vi "test Initial States Are Activated.vi"(8 "error in (no error)":errorcluster, 11 "TestCase in":refnum<class "Routing and Faulting System Tests.lvclass">) -> (0 "error out":errorcluster, 3 "TestCase out":refnum<class "Routing and Faulting System Tests.lvclass">)   [LabVIEW 2017, in "Routing and Faulting System Tests.lvclass"]
uses:
  Routing and Faulting System Tests.lvclass
  C:/Dev/GitHub/niveristand-custom-device-testing-tools/VeriStandTestCase/VeriStandTestCase.lvclass
  SLSC Switch States.ctl
  Routing and Faulting System Tests.lvclass/Routing and Faulting System Tests.ctl
  <vilib>/NI Veristand/Execution/Workspace/NI VeriStand - Get Single Channel Value.vi
  <vilib>/NI VeriStand/Execution/Workspace/NI_VS Workspace ExecutionAPI.lvlib
  <vilib>/addons/_JKI Toolkits/VI Tester/TestCase.llb/TestCase.lvclass
  C:/Program Files (x86)/National Instruments/LabVIEW 2017/vi.lib/addons/_JKI Toolkits/VI Tester/TestCase.llb/TestCase.lvclass
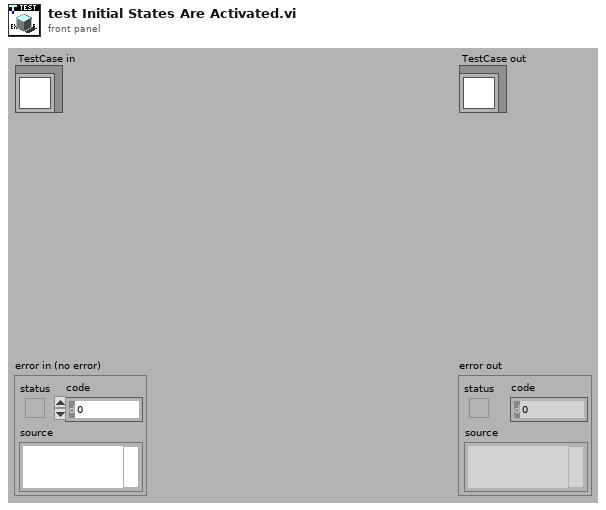
[diagram p1: front panel]
types:
  T1 = typedef "Routing and Faulting System Tests.lvclass/SLSC Switch States.ctl" = cluster{"Channel Load States":cluster{"name":string, "value":i32}[], "Channel Bus States":cluster{"name":string, "value":i32}[], "Channel Pair States":cluster{"name":string, "value":i32}[]}
  T2 = typedef "NI_VS Workspace ExecutionAPI.lvlib/WorkspaceAPI.ctl" = refnum<k24>
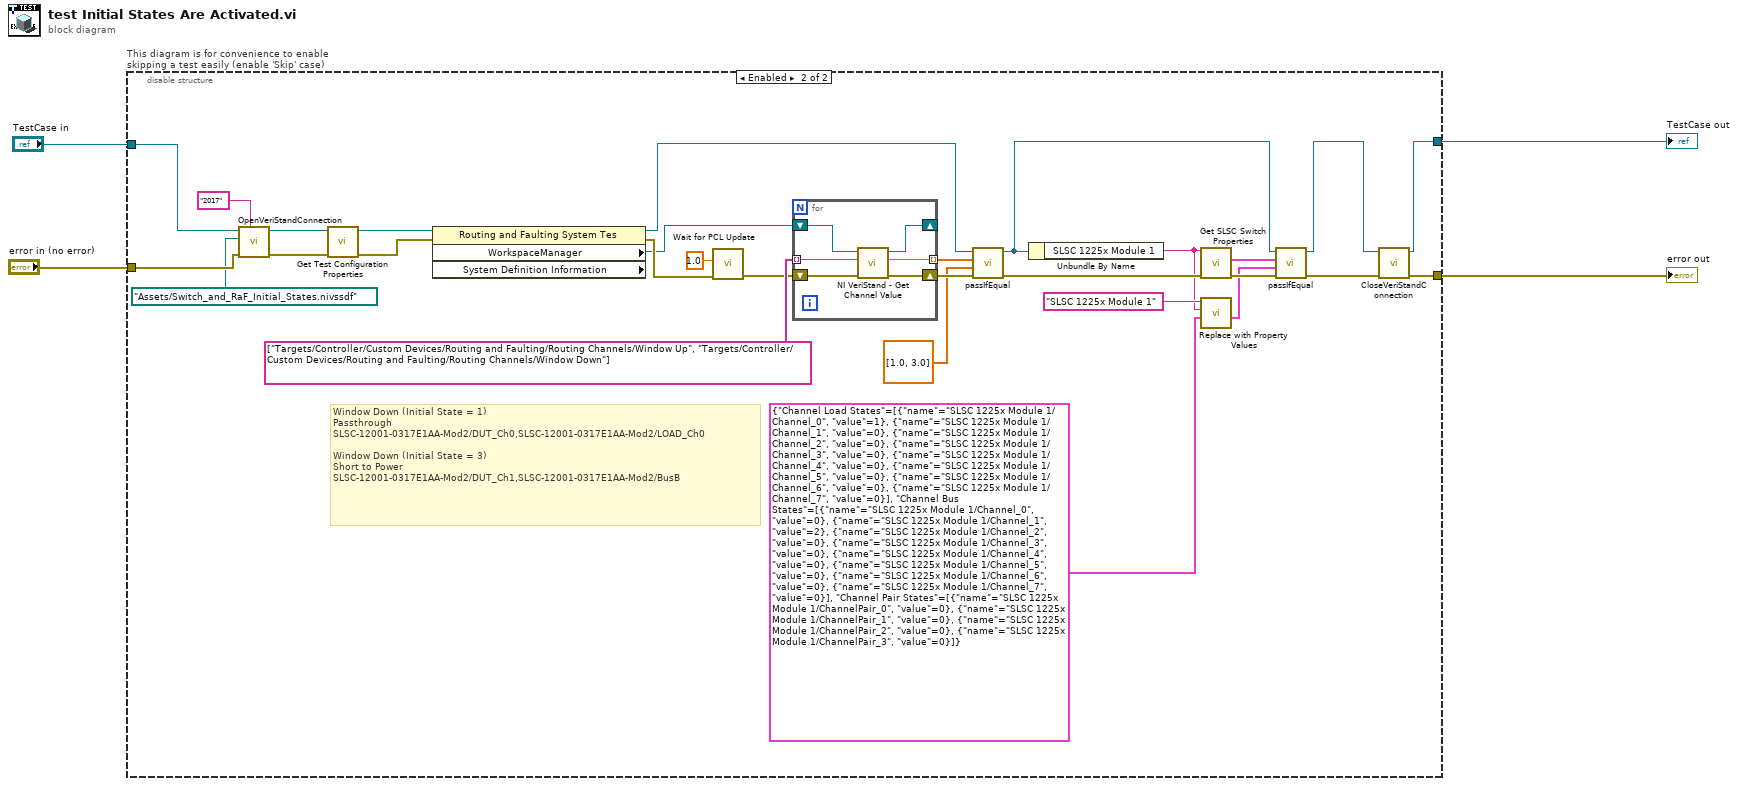
[diagram p0: block diagram]
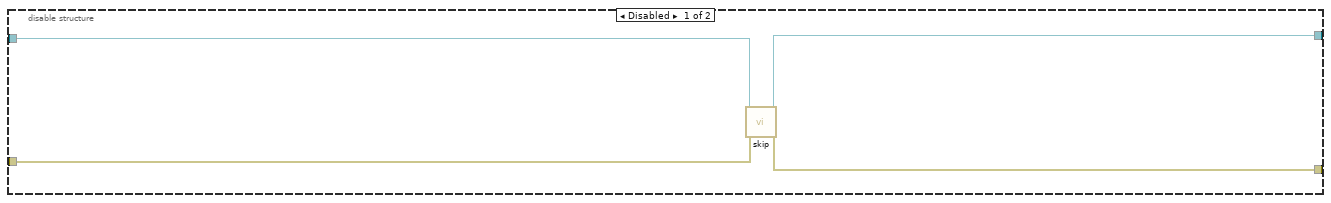
[diagram p2: hidden frame]
diagram:
  n1 = disable-structure "This diagram is for convenience to enable skipping a test easily (enable 'Skip' case)" shown="Enabled" {
    disable-tunnel: "TestCase in" -> [w8 w18]
    disable-tunnel: [w7 w26] -> w2
    disable-tunnel: [w6 w24] -> w1
    disable-tunnel: "error in (no error)" -> [w5 w36]
    frame Disabled {
      n2 = call <vilib>:"skip.vi"("error in (no error)"=w5, "TestCase in"=w8) -> ("error out"=w6:errorcluster, "TestCase out"=w7:refnum<class "Routing and Faulting System Tests.lvclass">)  [unwired: 8 in]
    }
    frame Enabled {
      # "Window Down (Initial State = 1)\nPassthrough\nSLSC-12001-0317E1AA-Mod2/DUT_Ch0,SLSC-12001-0317E1AA-Mod2/LOAD_Ch0\n\nWindow Down (Initial State = 3)\nShort to Power\nSLSC-12001-0317E1AA-Mod2/DUT_Ch1,SLSC-12001-0317E1AA-Mod2/BusB"
      n3 = call-dynamic "OpenVeriStandConnection.vi"("Minimum VeriStand Version (2016)"="2017" ("Minimum VeriStand Version (2015)"), "error in (no error)"=w36, "System Definition File"=path "Assets/Switch_and_RaF_Initial_States.nivssdf", "VeriStand Test Case in"=w18) -> ("error out"=w17:errorcluster, "VeriStand Test Case out"=w15:refnum<class "Routing and Faulting System Tests.lvclass">)  [unwired: 5 in, 1 out]
      n4 = call "Get Test Configuration Properties.vi"("error in (no error)"=w17, "Routing and Faulting System Tests in"=w15) -> ("error out"=w16:errorcluster, "Routing and Faulting System Tests out"=w14:refnum<class "Routing and Faulting System Tests.lvclass">)  [unwired: 8 in]
      n5 = property class="Routing and Faulting System Tes" props=["WorkspaceManager", "System Definition Information"](reference=w14, error in=w16) -> (reference out=w19:refnum<class "Routing and Faulting System Tests.lvclass">, error out=w22:errorcluster, "WorkspaceManager"=w20:T2)  [unwired: 1 out]
      n6 = call "Wait for PCL Update"("error in (no error)"=w22, "Delay Time (s)"=1.0) -> ("error out"=w21:errorcluster)  [unwired: 9 in]
      n7 = for {
        tunnel: [w41] -> w31 mode=indexing
        shift-right: [w39] -> w33
        shift-left: w21 -> [w43]
        shift-right: [w40] -> _
        shift-left: w20 -> [w42]
        tunnel: string[] ["Targets/Controller/Custom Devices/Routing and Faulting/Routing Channels/Window Up", "Targets/Controller/Custom Devices/Routing and Faulting/Routing Channels/Window Down"] -> [w38] mode=indexing
        n8 = call-poly <vilib>:"NI VeriStand - Get Channel Value.vi"("error in (no error)"=w43, "Channel"=w38, "WorkspaceManager in"=w42) -> ("error out"=w39:errorcluster, "Value"=w41:dbl, "WorkspaceManager out"=w40:T2)  [unwired: 6 in]
      }
      n9 = call-dynamic "passIfEqual.vi"("error in (no error)"=w33, "y"=dbl[] [1.0, 3.0], "x"=w31, "TestCase in"=w19) -> ("error out"=w32:errorcluster, "TestCase out"=w13:refnum<class "Routing and Faulting System Tests.lvclass">)  [unwired: 6 in]
      n10 = Unbundle By Name(w13) -> ("SLSC 1225x Module 1"=w11:string)
      n11 = call "Get SLSC Switch Properties.vi"("error in (no error)"=w32, "device"=w11) -> ("error out"=w29:errorcluster, "SLSC Switch States"=w28:T1)  [unwired: 8 in]
      n12 = call "Replace with Property Values.vi"("SLSC Switch States in"=T1 {"Channel Load States"=[{"name"="SLSC 1225x Module 1/Channel_0", "value"=1}, {"name"="SLSC 1225x Module 1/Channel_1", "value"=0}, {"name"="SLSC 1225x Module 1/Channel_2", "value"=0}, {"name"="SLSC 1225x Module 1/Channel_3", "value"=0}, {"name"="SLSC 1225x Module 1/Channel_4", "value"=0}, {"name"="SLSC 1225x Module 1/Channel_5", "value"=0}, {"name"="SLSC 1225x Module 1/Channel_6", "value"=0}, {"name"="SLSC 1225x Module 1/Channel_7", "value"=0}], "Channel Bus States"=[{"name"="SLSC 1225x Module 1/Channel_0", "value"=0}, {"name"="SLSC 1225x Module 1/Channel_1", "value"=2}, {"name"="SLSC 1225x Module 1/Channel_2", "value"=0}, {"name"="SLSC 1225x Module 1/Channel_3", "value"=0}, {"name"="SLSC 1225x Module 1/Channel_4", "value"=0}, {"name"="SLSC 1225x Module 1/Channel_5", "value"=0}, {"name"="SLSC 1225x Module 1/Channel_6", "value"=0}, {"name"="SLSC 1225x Module 1/Channel_7", "value"=0}], "Channel Pair States"=[{"name"="SLSC 1225x Module 1/ChannelPair_0", "value"=0}, {"name"="SLSC 1225x Module 1/ChannelPair_1", "value"=0}, {"name"="SLSC 1225x Module 1/ChannelPair_2", "value"=0}, {"name"="SLSC 1225x Module 1/ChannelPair_3", "value"=0}]} ("SLSC Switch States"), "replace string"=w11, "search string"="SLSC 1225x Module 1" ("name")) -> ("SLSC Switch States out"=w9:T1)  [unwired: 8 in]
      n13 = call-dynamic "passIfEqual.vi"("error in (no error)"=w29, "y"=w9, "x"=w28, "TestCase in"=w13) -> ("error out"=w25:errorcluster, "TestCase out"=w27:refnum<class "Routing and Faulting System Tests.lvclass">)  [unwired: 6 in]
      n14 = call-dynamic "CloseVeriStandConnection.vi"("error in (no error)"=w25, "VeriStand Test Case in"=w27) -> ("error out"=w24:errorcluster, "VeriStand Test Case out"=w26:refnum<class "Routing and Faulting System Tests.lvclass">)  [unwired: 8 in]
    }
  }
  "error out" <- w1
  "TestCase out" <- w2
